vi "UiSchematic.vi"() -> ()   [LabVIEW 2011]
uses:
  Tank.ctl
  VentilS.ctl
  Pumpe.ctl
  MR.ctl
  VentilW.ctl
  Output - Cluster b2g1.ctl
  Output - Cluster b2g2.ctl
  <vilib>/Platform/TimedLoop/XDataNode/timing_clust.ctl
  <vilib>/Platform/TimedLoop/XDataNode/nitl_modes.ctl
  <vilib>/Platform/TimedLoop/XDataNode/wakeup.ctl
  <vilib>/Platform/TimedLoop/XDataNode/XDataNode.xnode
  <vilib>/Platform/TimedLoop/XDataNode/XDNodeRunTimeDep.lvlib
panel:
  out "T-2 Min!":bool
  out "T-2 Max!":bool
  in  "Output Var B2G2":refnum<k21>="ni.var.psp://10.27.40.21/variables - b2g2/data - network b2g2"
  out "V-14":T1
  out "V-33":T2
  out "V-34":T2
  out "V-35":T2
  out "V-10":T2
  out "P-4 [%] 2":u8
  out "P-4 ERR":bool
  out "P-4":T3
  out "DFS-1 [dl]":u64
  out "DFS-1 [l/min]":dbl format="%.2f"
  out "HS-1":bool
  out "HS-1":bool
  out "TS-5 [°C]":dbl format="%.2g"
  out "pHS-1 [pH] 2":dbl format="%.2g"
  out "TS-4 [°C]":dbl format="%.2g"
  out "DS-1 [bar]":dbl format="%.2g"
  out "B2G2 V-15":u8
  out "V-15":T2
  out "V-13":u8
  out "V-13":T2
  out "MR Min! 2":bool
  out "MR Max! 2":bool
  out "B2G2 FS-2 [l]":T4 scale=10.0..80.0 scale format="%#.2g"
  out "B2G2 FS-3 [l]":T5 scale=0.0..5.0 scale format="%#.1g"
  in  "Output Var B2G1":refnum<k21>="ni.var.psp://10.27.40.24/variables - b2g1/data - network - b2g1"
  in  "stop":bool
  out "P-4 ERR":bool
  out "P-5 ERR":bool
  out "TS-5 [°C]":dbl format="%.2g"
  out "HS-1 2":bool
  out "P-4":T3
  out "DFS-1 [dl]":u64
  out "DFS-1 [l/min]":dbl format="%.2f"
  out "P-4 [%]":u8
  out "P-5 [%]":u8
  out "V-14":T2
  out "V-33":T2
  out "HS-1":bool
  out "pHS-1 [pH]":dbl format="%.2g"
  out "TS-4 [°C]":dbl format="%.2g"
  out "DS-1 [bar]":dbl format="%.2g"
  out "V-13":u8
  out "V-15":u8
  out "V-13":T2
  out "P-5":T3
  out "T-2 Max!":bool
  out "T-2 Min!":bool
  out "T-1 Min!":bool
  out "T-1 Max!":bool
  out "V-15":T2
  out "V-10":T2
  out "MR Min!":bool
  out "MR Max!":bool
  out "V-34":T2
  out "B2G1 FS-1 [l]":T4 scale=10.0..80.0 scale format="%#.2g"
  out "B2G1 FS-2 [l]":T4 scale=10.0..80.0 scale format="%#.2g"
  out "B2G1 FS-3 [l]":T5 scale=0.0..5.0 scale format="%#.1g"
  # "T-2"
  # "T-2"
  # "B2G1"
  # "B2G2"
  # "T-1"
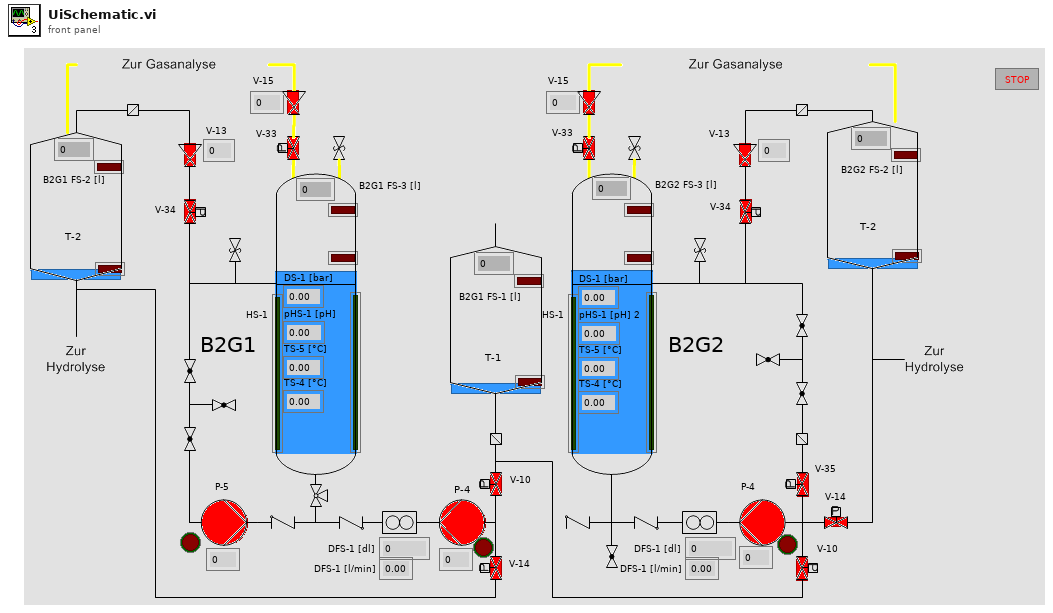
[diagram p1: front panel]
types:
  T1 = typedef "VentilW.ctl" = bool
  T2 = typedef "VentilS.ctl" = bool
  T3 = typedef "Pumpe.ctl" = bool
  T4 = typedef "Tank.ctl" = dbl
  T5 = typedef "MR.ctl" = dbl
  T6 = typedef "Output - Cluster b2g2.ctl" = cluster{"DFS-1 [dl]":u64, "FS-3 [l]":dbl, "DFS-1 [l/min]":dbl, "DS-1 [bar]":dbl, "V-10 ZU":bool, "V-14 ZU":bool, "FS-1 [l]":dbl, "FS-2 [l]":dbl, "TS-4 [°C]":dbl, "HS-1":bool, "V-13 [%]":u8, "V-15 [%]":u8, "P-4 [%]":u8, "Dosierung":bool, "MR Max Füllstand":bool, "MR Min Füllstand":bool, "Dosiermenge [l]":sgl, "V-14 AUF":bool, "V-10 AUF":bool, "T-1 Max Füllstand":bool, "T-1 Min Füllstand":bool, "T-2 Max Füllstand":bool, "T-2 Min Füllstand":bool, "pHS-1 [pH]":dbl, "P-4 RUN":bool, "V-33 AUF":bool, "V-33 ZU":bool, "V-34 AUF":bool, "V-34 ZU":bool, "P-4 ERR":bool, "TS-5 [°C]":dbl, "V-35 AUF":bool, "V-35 ZU":bool}
  T7 = typedef "Output - Cluster b2g1.ctl" = cluster{"DFS-1 [dl]":u64, "FS-3 [l]":dbl, "DFS-1 [l/min]":dbl, "DS-1 [bar]":dbl, "V-10 ZU":bool, "V-14 ZU":bool, "FS-1 [l]":dbl, "FS-2 [l]":dbl, "TS-4 [°C]":dbl, "HS-1":bool, "V-13 [%]":u8, "V-15 [%]":u8, "P-4 [%]":u8, "P-5 [%]":u8, "Dosierung":bool, "MR Max Füllstand":bool, "MR Min Füllstand":bool, "Dosiermenge [l]":sgl, "V-14 AUF":bool, "V-10 AUF":bool, "T-1 Max Füllstand":bool, "T-1 Min Füllstand":bool, "T-2 Max Füllstand":bool, "T-2 Min Füllstand":bool, "pHS-1 [pH]":dbl, "P-4 RUN":bool, "P-5 RUN ":bool, "V-33 AUF":bool, "V-33 ZU":bool, "V-34 AUF":bool, "V-34 ZU":bool, "P-4 ERR":bool, "P-5 ERR":bool, "TS-5 [°C]":dbl, "GZ-1 [dl]":u64, "TS-6 [°C]":dbl, "DS-3 [bar]":dbl}
  T8 = typedef "XDNodeRunTimeDep.lvlib/timing_clust.ctl" = cluster{"Expected End [f-1]":u64, "Actual End [f-1]":u64, "Finished Late? [f-1]":bool, "Expected End [i-1]":u64, "Actual End [i-1]":u64, "Finished Late? [i-1]":bool, "Expected Start [i]":u64, "Actual Start [i]":u64, "Expected Start [f]":u64, "Actual Start [f]":u64, "Source Name":string, "Structure Name":string, "Period":i64, "Deadline":i64, "Offset":i64, "Start":i64, "Priority":i32, "Timeout":i32, "Mode":T9, "Wakeup Reason":T10, "Error":errorcluster, "Source Type":string, "Secondary Source Type":string, "Global End Time":u64, "Global Start Time":u64, "Frame Duration":u64, "Iteration Duration":u64, "Assigned CPU":i32, "I/O Scan Engine Mode":u32}
  T9 = typedef "XDNodeRunTimeDep.lvlib/nitl_modes.ctl" = enum32{"No Change", "Process missed periods, maintain original phase", "Discard missed periods, maintain original phase", "Process missed periods, ignore original phase", "Discard missed periods, ignore original phase"}
  T10 = typedef "XDNodeRunTimeDep.lvlib/wakeup.ctl" = enum32{"Normal", "Aborted", "Asynchronous wakeup", "Timing source error", "Timed loop error", "Timeout"}
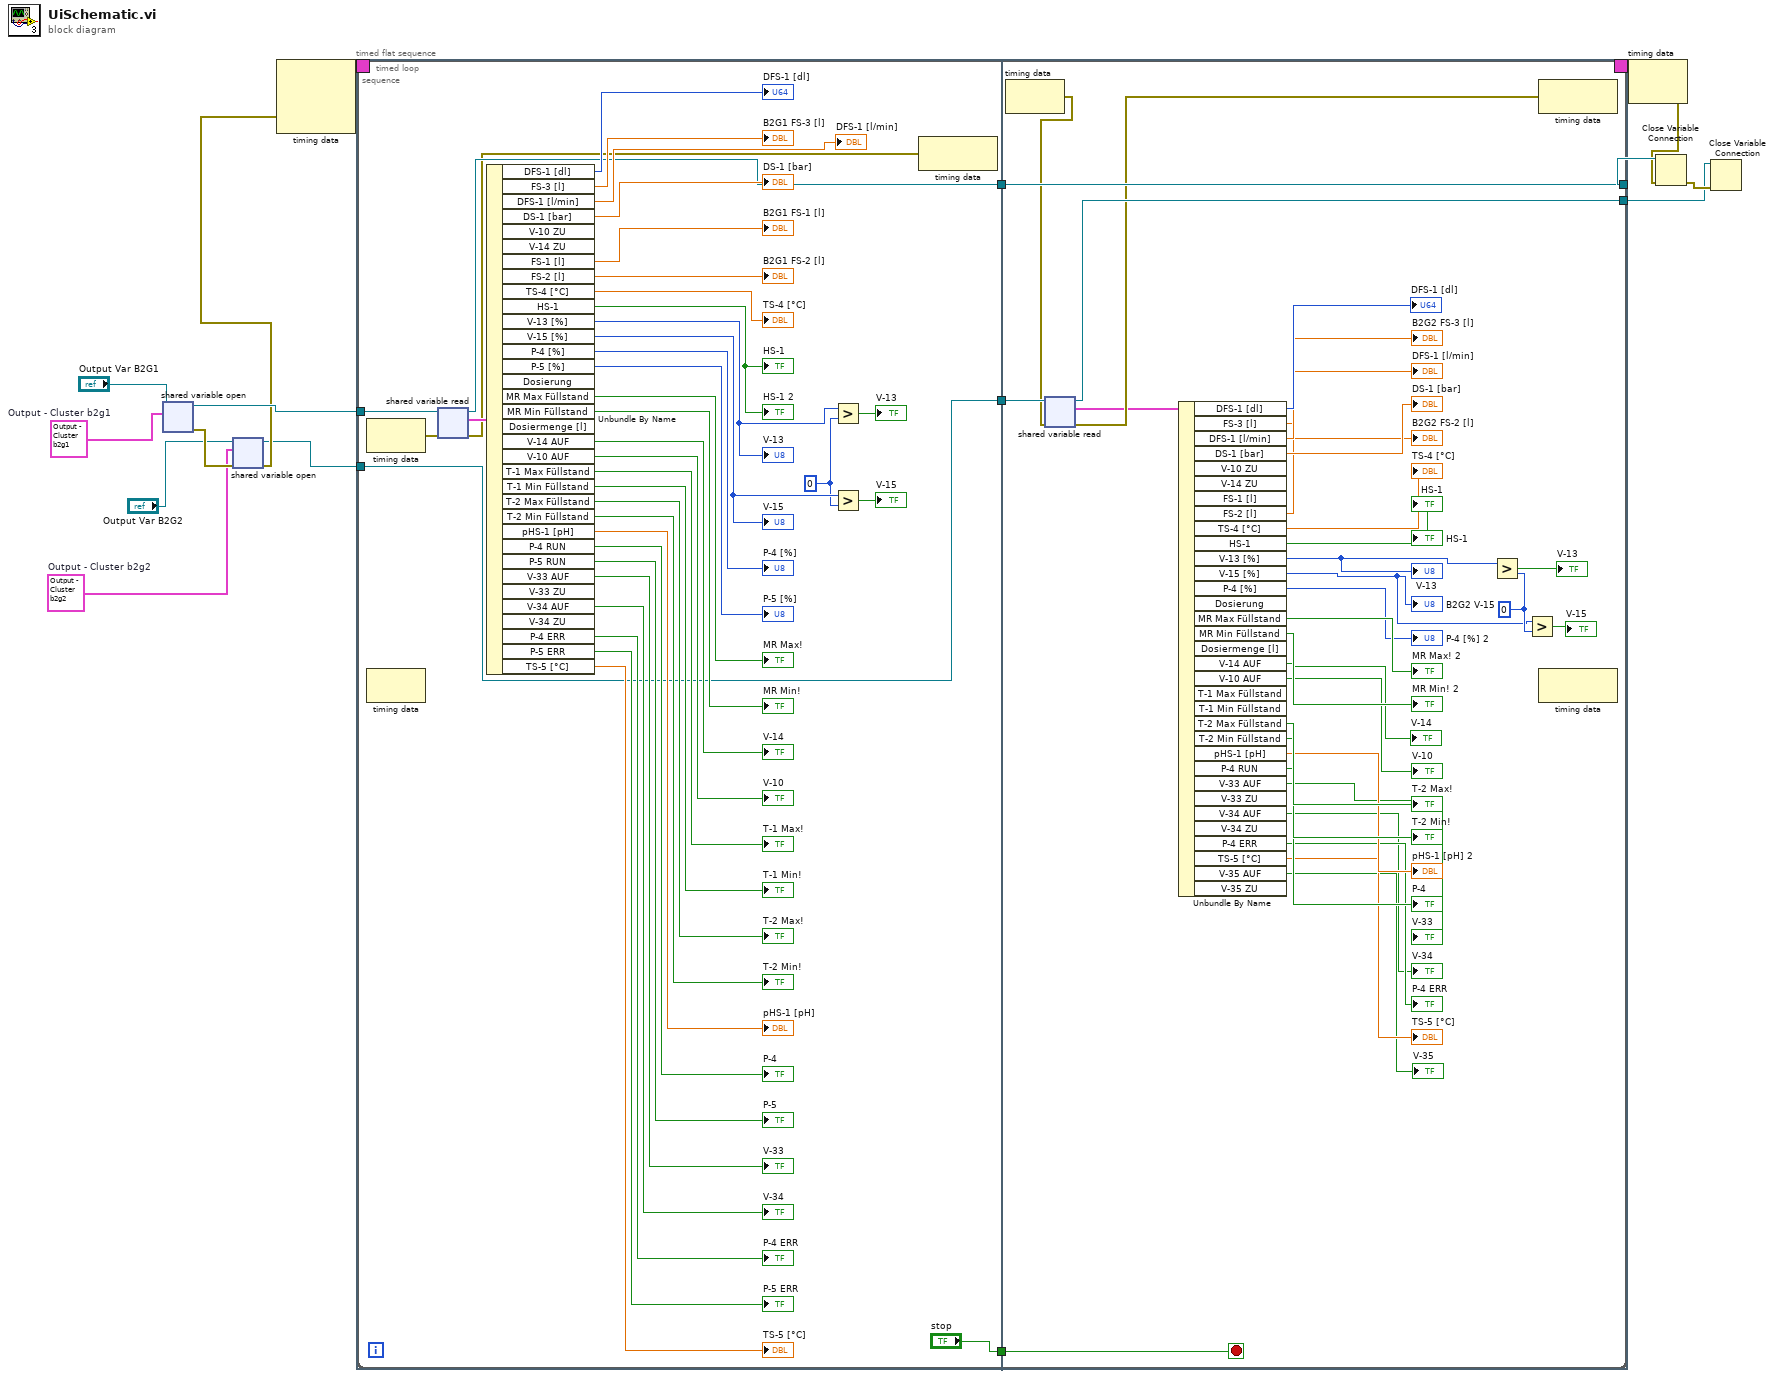
[diagram p0: block diagram]
diagram:
  w2 = T6 {"DFS-1 [dl]"=0, "FS-3 [l]"=0.0, "DFS-1 [l/min]"=0.0, "DS-1 [bar]"=0.0, "V-10 ZU"=FALSE, "V-14 ZU"=FALSE, "FS-1 [l]"=0.0, "FS-2 [l]"=0.0, "TS-4 [°C]"=0.0, "HS-1"=FALSE, "V-13 [%]"=0, "V-15 [%]"=0, "P-4 [%]"=0, "Dosierung"=FALSE, "MR Max Füllstand"=FALSE, "MR Min Füllstand"=FALSE, "Dosiermenge [l]"=0.0, "V-14 AUF"=FALSE, "V-10 AUF"=FALSE, "T-1 Max Füllstand"=FALSE, "T-1 Min Füllstand"=FALSE, "T-2 Max Füllstand"=FALSE, "T-2 Min Füllstand"=FALSE, "pHS-1 [pH]"=0.0, "P-4 RUN"=FALSE, "V-33 AUF"=FALSE, "V-33 ZU"=FALSE, "V-34 AUF"=FALSE, "V-34 ZU"=FALSE, "P-4 ERR"=FALSE, "TS-5 [°C]"=0.0, "V-35 AUF"=FALSE, "V-35 ZU"=FALSE}  # Output - Cluster b2g2
  w12 = T7 {"DFS-1 [dl]"=0, "FS-3 [l]"=0.0, "DFS-1 [l/min]"=0.0, "DS-1 [bar]"=0.0, "V-10 ZU"=FALSE, "V-14 ZU"=FALSE, "FS-1 [l]"=0.0, "FS-2 [l]"=0.0, "TS-4 [°C]"=0.0, "HS-1"=FALSE, "V-13 [%]"=0, "V-15 [%]"=0, "P-4 [%]"=0, "P-5 [%]"=0, "Dosierung"=FALSE, "MR Max Füllstand"=FALSE, "MR Min Füllstand"=FALSE, "Dosiermenge [l]"=0.0, "V-14 AUF"=FALSE, "V-10 AUF"=FALSE, "T-1 Max Füllstand"=FALSE, "T-1 Min Füllstand"=FALSE, "T-2 Max Füllstand"=FALSE, "T-2 Min Füllstand"=FALSE, "pHS-1 [pH]"=0.0, "P-4 RUN"=FALSE, "P-5 RUN "=FALSE, "V-33 AUF"=FALSE, "V-33 ZU"=FALSE, "V-34 AUF"=FALSE, "V-34 ZU"=FALSE, "P-4 ERR"=FALSE, "P-5 ERR"=FALSE, "TS-5 [°C]"=0.0, "GZ-1 [dl]"=0, "TS-6 [°C]"=0.0, "DS-3 [bar]"=0.0}  # Output - Cluster b2g1
  n1 = shared-variable-open("Output Var B2G1", w12) -> (w13:refnum<k21>, w5:errorcluster)  [unwired: 2 in]
  n2 = shared-variable-open("Output Var B2G2", w5, w2) -> (w1:refnum<k21>, w4:errorcluster)  [unwired: 1 in]
  n3 = node-c288(w4) -> (w10:T8)  [unwired: 2 in]
  n4 = timed-loop {
    timing: w10 -> [_]
    timing-out: [_] -> w9
    tunnel: w13 -> [w18]
    tunnel: [w17] -> w11
    tunnel: [w16] -> w6
    tunnel: w1 -> [w15]
    stop <- w100 stop-if-true
    n5 = timed-sequence {
      timing: _ -> [_]
      timing-out: _ -> [_]
      tunnel: w18 -> [w25]
      tunnel: [w24] -> w17
      tunnel: [w21] -> w16
      tunnel: w15 -> [w19]
      n6 = timed-flat-sequence {
        tunnel: w25 -> [w35]
        tunnel: [w33] -> w23
        tunnel: ["stop"] -> w22
        tunnel: [w26] -> w20
        tunnel: w19 -> [w26]
        tunnel: [w101] -> w24
        tunnel: w23 -> [w101]
        tunnel: w22 -> [w100]
        tunnel: [w99] -> w21
        tunnel: w20 -> [w98]
        frame #0 {
          w40 = u8 0 ("y")
          n7 = node-c288() -> (w32:errorcluster)  [unwired: 1 in]
          n8 = shared-variable-read(w35, w32) -> (w33:refnum<k21>, w31:errorcluster, w34:T7)  [unwired: 1 out]
          n9 = Unbundle By Name(w34) -> ("DFS-1 [dl]"=→"DFS-1 [dl]":u64, "FS-3 [l]"=→"B2G1 FS-3 [l]":dbl, "DFS-1 [l/min]"=→"DFS-1 [l/min]":dbl, "DS-1 [bar]"=→"DS-1 [bar]":dbl, "FS-1 [l]"=→"B2G1 FS-1 [l]":dbl, "FS-2 [l]"=→"B2G1 FS-2 [l]":dbl, "TS-4 [°C]"=→"TS-4 [°C]":dbl, "HS-1"=→"HS-1" →"HS-1 2":bool, "V-13 [%]"=w39:u8, "V-15 [%]"=w41:u8, "P-4 [%]"=→"P-4 [%]":u8, "P-5 [%]"=→"P-5 [%]":u8, "MR Max Füllstand"=→"MR Max!":bool, "MR Min Füllstand"=→"MR Min!":bool, "V-14 AUF"=→"V-14":bool, "V-10 AUF"=→"V-10":bool, "T-1 Max Füllstand"=→"T-1 Max!":bool, "T-1 Min Füllstand"=→"T-1 Min!":bool, "T-2 Max Füllstand"=→"T-2 Max!":bool, "T-2 Min Füllstand"=→"T-2 Min!":bool, "pHS-1 [pH]"=→"pHS-1 [pH]":dbl, "P-4 RUN"=→"P-4":bool, "P-5 RUN"=→"P-5":bool, "V-33 AUF"=→"V-33":bool, "V-34 AUF"=→"V-34":bool, "P-4 ERR"=→"P-4 ERR":bool, "P-5 ERR"=→"P-5 ERR":bool, "TS-5 [°C]"=→"TS-5 [°C]":dbl)  [unwired: 6 out]
          "V-15" <- w41
          "V-13" <- w39
          n10 = Greater?(x=w39, y=w40) -> (0:→"V-13":bool)
          n11 = Greater?(x=w41, y=w40) -> (0:→"V-15":bool)
          n12 = node-c288(w31) -> ()  [unwired: 1 out]
        }
        frame #1 {
          w79 = u8 0 ("y")
          n13 = node-c288() -> (w97:errorcluster)  [unwired: 1 in]
          n14 = shared-variable-read(w98, w97) -> (w99:refnum<k21>, w96:errorcluster, w95:T6)  [unwired: 1 out]
          n15 = Unbundle By Name(w95) -> ("DFS-1 [dl]"=→"DFS-1 [dl]":u64, "FS-3 [l]"=→"B2G2 FS-3 [l]":dbl, "DFS-1 [l/min]"=→"DFS-1 [l/min]":dbl, "DS-1 [bar]"=→"DS-1 [bar]":dbl, "FS-2 [l]"=→"B2G2 FS-2 [l]":dbl, "TS-4 [°C]"=→"TS-4 [°C]":dbl, "HS-1"=→"HS-1" →"HS-1":bool, "V-13 [%]"=w71:u8, "V-15 [%]"=w78:u8, "P-4 [%]"=→"P-4 [%] 2":u8, "MR Max Füllstand"=→"MR Max! 2":bool, "MR Min Füllstand"=→"MR Min! 2":bool, "V-14 AUF"=→"V-14":bool, "V-10 AUF"=→"V-10":bool, "T-2 Max Füllstand"=→"T-2 Max!":bool, "T-2 Min Füllstand"=→"T-2 Min!":bool, "pHS-1 [pH]"=→"pHS-1 [pH] 2":dbl, "P-4 RUN"=→"P-4":bool, "V-33 AUF"=→"V-33":bool, "V-34 AUF"=→"V-34":bool, "P-4 ERR"=→"P-4 ERR":bool, "TS-5 [°C]"=→"TS-5 [°C]":dbl, "V-35 AUF"=→"V-35":bool)  [unwired: 10 out]
          "B2G2 V-15" <- w78
          "V-13" <- w71
          n16 = Greater?(x=w71, y=w79) -> (0:→"V-13":bool)
          n17 = Greater?(x=w78, y=w79) -> (0:→"V-15":bool)
          n18 = node-c288(w96) -> ()  [unwired: 1 out]
        }
      }
    }
    n19 = node-c288() -> ()  [unwired: 1 in, 1 out]
    n20 = node-c288() -> ()  [unwired: 1 in, 1 out]
  }
  n21 = node-c288(w9) -> (w8:errorcluster)
  n22 = Close Variable Connection(8:w8, 11:w11) -> (0:w7:errorcluster)
  n23 = Close Variable Connection(8:w7, 11:w6) -> ()  [unwired: 1 out]
